vi "Agilent SNA Set SRQ Mask.vi"(6 "Channel":i8=1 min=1 max=99 step=1, 7 "Agilent SNA & SWP":T1, 8 "error in (no error)":errorcluster, 10 "SRQ Mask":u8=255 format="%08b", 11 "VISA Resource Names":T2) -> (0 "error out":errorcluster, 3 "dup VISA Resource Names":T2)   [LabVIEW 2011]
doc: "This VI for the HP8753B Network Analyzers reads the stimulus values. Except when performing log sweeps and freq list sweeps, this VI uses the start and stop values and the number of points to calcuate the stimulus values."
uses:
  TypeDefs/Agilent SNA VISA.ctl
  TypeDefs/Agilent SNA Instrument Info.ctl
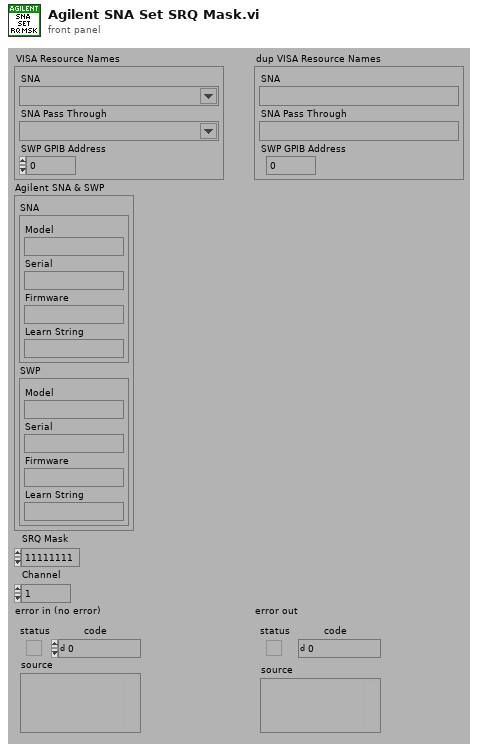
[diagram p1: front panel]
types:
  T1 = typedef "Agilent SNA Instrument Info.ctl" = cluster{"SNA":cluster{"Model":string, "Serial":string, "Firmware":string, "Learn String":string}, "SWP":cluster{"Model":string, "Serial":string, "Firmware":string, "Learn String":string}}
  T2 = typedef "Agilent SNA VISA.ctl" = cluster{"SNA":refnum<visa-resource-name>, "SNA Pass Through":refnum<visa-resource-name>, "SWP GPIB Address":i32}
  T3 = typedef "Agilent SNA Model.ctl" = enum16{"Not Supported", "8757X"}
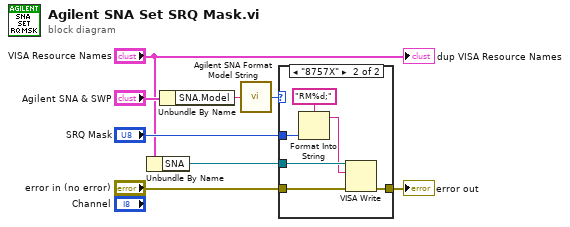
[diagram p0: block diagram]
diagram:
  n1 = Unbundle By Name("VISA Resource Names") -> ("SNA"=w4:refnum<visa-resource-name>)
  n2 = Unbundle By Name("Agilent SNA & SWP") -> ("SNA.Model"=w6:string)
  n3 = call "Agilent SNA Format Model String.vi"("Model String"=w6) -> ("Model"=w5:T3)
  n4 = case shown="\"8757X\"" w5 {
    tunnel: [w9 w13] -> w8
    tunnel: "SRQ Mask" -> [_ w10]
    tunnel: "error in (no error)" -> [w9 w15]
    tunnel: w4 -> [_ w14]
    frame "Not Supported" {
    }
    frame "8757X" {
      n5 = Format Into String(format string="RM%d;", w10) -> (resulting string=w11:string)  [unwired: 2 in, 1 out]
      n6 = VISA Write(VISA resource name=w14, write buffer=w11, error in (no error)=w15) -> (error out=w13:errorcluster)  [unwired: 2 out]
    }
  }
  "error out" <- w8
  "dup VISA Resource Names" <- "VISA Resource Names"
